vi "MouseButtonDown.vi"(4 "y":sgl, 5 "Clicks":u8, 6 "x":sgl, 7 "Button":u8, 8 "error in (no error)":errorcluster, 9 "Which":T1, 10 "Timestamp":u64, 11 "WindowEventInterface in":refnum<class "WindowEventInterface.lvclass">) -> (0 "error out":errorcluster)   [LabVIEW 2020, in "GLF.lvlib" / "WindowEventInterface.lvclass"]
uses:
  WindowEventInterface.lvclass
  <vilib>/Saukko/LV SDL3/Sources/SDL3/Mouse/MouseID--integer.ctl
  <vilib>/Saukko/LV SDL3/Sources/SDL3/Mouse/Mouse.lvlib
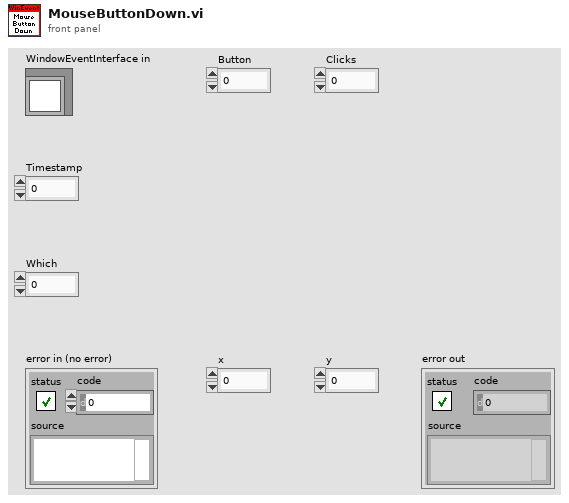
[diagram p1: front panel]
types:
  T1 = typedef "SDL3.lvlib/Mouse.lvlib/MouseID--integer.ctl" = u32
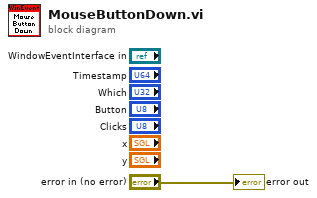
[diagram p0: block diagram]
diagram:
  "error out" <- "error in (no error)"
